vi "Event Next Frame.vi"(0 "Diagram in":refnum<vi>, 5 "Event Data Out Names":string[](array[string]), 7 "Event Data out":refnum<vi>[](array[refnum]), 9 "Event Data In Names":string[](array[string]), 11 "error in (no error)":errorcluster) -> (4 "Selected Diagram":refnum<vi>, 6 "Inputs":refnum<vi>[](array[refnum]), 8 "Event Data in":refnum<vi>[](array[refnum]), 15 "error out":errorcluster)   [LabVIEW 2015, in "Scripting.lvlib"]
doc: "Navigates to the next frame of the Event Structure that owns <B>Diagram in</B>, supplying the frame's diagram at <B>Diagram out</B>.\n\n<B>Event Data Out Names</B> are the names of the desired Event Data out elements of the current frame.\n\n<B>Event Data Out<B> is an array of terminals to wire to the configured Event Data out terminals.\n\n<B>Event Data in Names</B> are the names of the desired Event Data in elements of the next frame.\n\n<B>Event Data in</B> is an array containing the configured terminals of the Event Data in node of the next frame."
uses:
  Scripting.lvlib
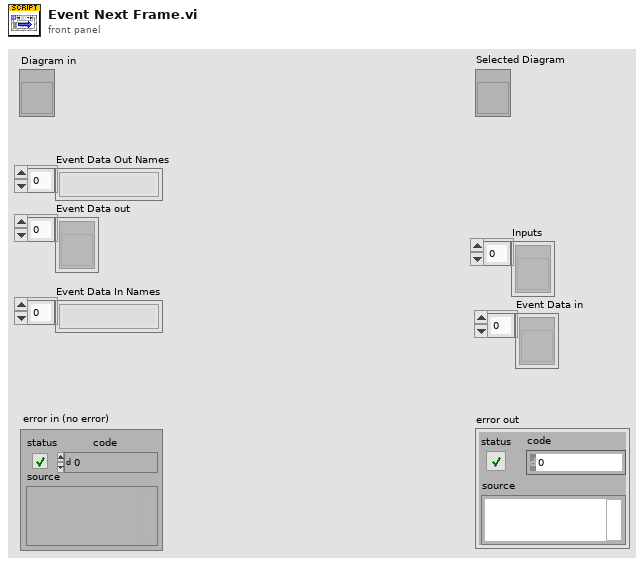
[diagram p1: front panel]
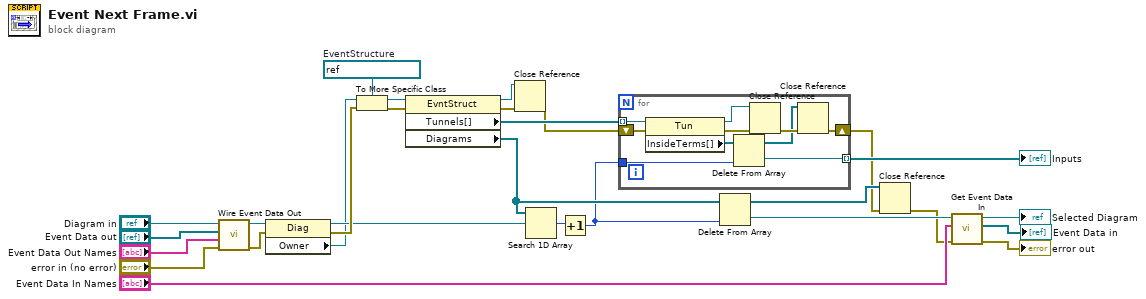
[diagram p0: block diagram]
diagram:
  w27 = refnum<vi> refnum  # EventStructure
  n1 = call "Wire Event Data Out.vi"("error in (no error)"="error in (no error)", "Event Data Names"="Event Data Out Names", "Event Data"="Event Data out", "Diagram in"="Diagram in") -> ("error out"=w14:errorcluster, "Diagram out"=w12:refnum<vi>)  [unwired: 6 in]
  n2 = property class="Diag"(reference=w12, error in=w14) -> (reference out=w11:refnum<vi>, error out=w13:errorcluster, "Owner"=w10:refnum<vi>)
  n3 = To More Specific Class(target class=w27, reference=w10, error in=w13) -> (specific class reference=w18:refnum<vi>, error out=w17:errorcluster)
  n4 = property class="EvntStruct"(reference=w18, error in=w17) -> (reference out=w4:refnum<vi>, error out=w19:errorcluster, "Tunnels[]"=w20:refnum<vi>[], "Diagrams"=w23:refnum<vi>[])
  n5 = Close Reference(reference=w4, error in (no error)=w19) -> (error out=w5:errorcluster)
  n6 = Search 1D Array(1D array=w23, element=w11) -> (index of element=w22:i32)  [unwired: 1 in]
  n7 = Increment(x=w22) -> (x+1=w21:i32)
  n8 = for {
    tunnel: w20 -> [w38] mode=indexing
    tunnel: w21 -> [w36]
    shift-right: [w30] -> w2
    shift-left: w5 -> [w35]
    tunnel: [w33] -> w26 mode=indexing
    n9 = property class="Tun"(reference=w38, error in=w35) -> (reference out=w31:refnum<vi>, error out=w34:errorcluster, "InsideTerms[]"=w37:refnum<vi>[])
    n10 = Delete From Array(array=w37, index=w36) -> (deleted portion=w33:refnum<vi>, array with subset deleted=w29:refnum<vi>[])  [unwired: 1 in]
    n11 = Close Reference(reference=w31, error in (no error)=w34) -> (error out=w32:errorcluster)
    n12 = Close Reference(reference=w29, error in (no error)=w32) -> (error out=w30:errorcluster)
  }
  "Inputs" <- w26
  n13 = Delete From Array(array=w23, index=w21) -> (deleted portion=w28:refnum<vi>, array with subset deleted=w3:refnum<vi>[])  [unwired: 1 in]
  n14 = Close Reference(reference=w3, error in (no error)=w2) -> (error out=w1:errorcluster)
  n15 = call "Get Event Data In.vi"("error in (no error)"=w1, "Event Data Names"="Event Data In Names", "Diagram in"=w28) -> ("error out"=→"error out":errorcluster, "OutputTerms[]"=→"Event Data in":refnum<vi>[], "Diagram out"=→"Selected Diagram":refnum<vi>)  [unwired: 6 in]
